vi "RSZVB Set Hold.vi"(8 "error in (no error)":errorcluster {"code" format="%.0x"}, 9 "Hold (1)":i32(ring)=1 items=["Off", "Max", "Min"], 10 "Channel (1)":i32=1, 11 "VISA session":refnum<visa-resource-name>) -> (0 "error out":errorcluster {"code" format="%.0x"}, 3 "dup VISA session":refnum<visa-resource-name>)   [LabVIEW 2011]
doc: "This VI enables, disables, or restarts the max hold and the min hold VIs \n\nRemote-control command(s):\nCALCulate<Chn>:PHOLd MIN | MAX | OFF"
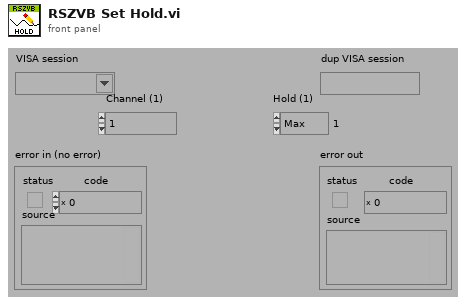
[diagram p1: front panel]
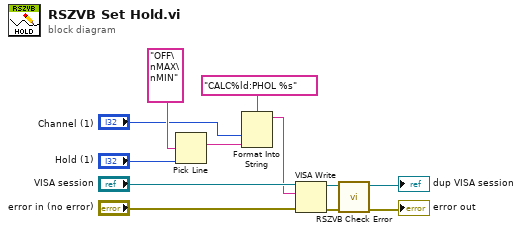
[diagram p0: block diagram]
diagram:
  n1 = Pick Line(multi-line string="OFF\nMAX\nMIN", line index="Hold (1)") -> (output string=w8:string)  [unwired: 1 in]
  n2 = Format Into String(format string="CALC%ld:PHOL %s", "Channel (1)", w8) -> (resulting string=w5:string)  [unwired: 2 in, 1 out]
  n3 = VISA Write(VISA resource name="VISA session", write buffer=w5, error in (no error)="error in (no error)") -> (VISA resource name out=w3:refnum<visa-resource-name>, error out=w4:errorcluster)  [unwired: 1 out]
  n4 = call "RSZVB Check Error.vi"("error in (no error)"=w4, "VISA session"=w3) -> ("error out"=→"error out":errorcluster, "dup VISA session"=→"dup VISA session":refnum<visa-resource-name>)  [unwired: 8 in]
